vi "Coord list setup-format and values.vi"() -> (13 "Values.Boolean":bool[](array[boolean]), 14 "Keys setup.DBL":T2=[{"key"="Control FPGA.Clock Freq (MHz)", "Save?"=TRUE, "Default"=240.0}, {"key"="DAQ FPGA.Clock Freq (MHz)", "Save?"=TRUE, "Default"=240.0}], 15 "Values.DBL":dbl[](array[numeric]) format="%#_9f", 16 "Keys setup.String":T3=[{"key"="Control FPGA.MAC address", "Save?"=TRUE, "Default"="AABBCCDDEEFF"}, {"key"="DAQ FPGA.Target", "Save?"=TRUE, "Default"="RIO0"}, {"key"="XY Stage.COM port", "Save?"=TRUE, "Default"="COM7"}, {"key"="DAQmx Chan.Pockels Control", "Save?"=TRUE, "Default"=""}, {"key"="DAQmx Chan.Hard Shutter", "Save?"=TRUE, "Default"=""}, {"key"="DAQmx Chan.PMT 1", "Save?"=TRUE, "Default"=""}, {"key"="DAQmx Chan.PMT 2", "Save?"=TRUE, "Default"=""}, {"key"="DAQmx Chan.Encoder Trigger", "Save?"=TRUE, "Default"=""}, {"key"="DAQmx Chan.Optional Trigger 1", "Save?"=TRUE, "Default"=""}, {"key"="DAQmx Chan.Optional Trigger 2", "Save?"=TRUE, "Default"=""}, {"key"="DAQmx Chan.Optional Trigger 3", "Save?"=TRUE, "Default"=""}], 17 "Values.Strings":string[](array[string]), 18 "Keys setup.Boolean":T1, 19 "error out":errorcluster)   [LabVIEW 2017]
uses:
  Typedefs/Ini file interface (String).ctl
  Typedefs/Ini file interface (DBL).ctl
  Typedefs/Ini file interface (Boolean).ctl
  User Interface/Windows/Coordinates list window/Globals/Coord window-Globals.vi
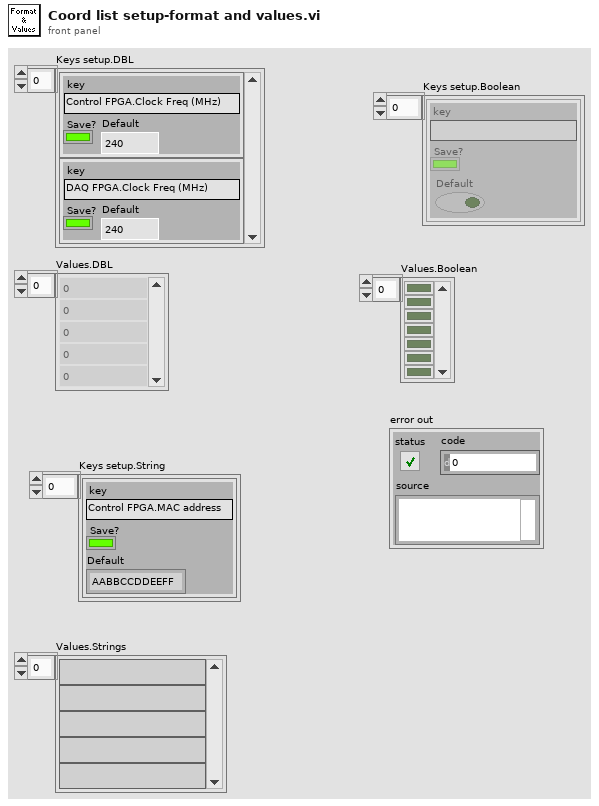
[diagram p1: front panel]
types:
  T1 = typedef "Ini file interface (Boolean).ctl" = cluster{"key":string, "Save?":bool, "Default":bool}[]
  T2 = typedef "Ini file interface (DBL).ctl" = cluster{"key":string, "Save?":bool, "Default":dbl}[]
  T3 = typedef "Ini file interface (String).ctl" = cluster{"key":string, "Save?":bool, "Default":string}[]
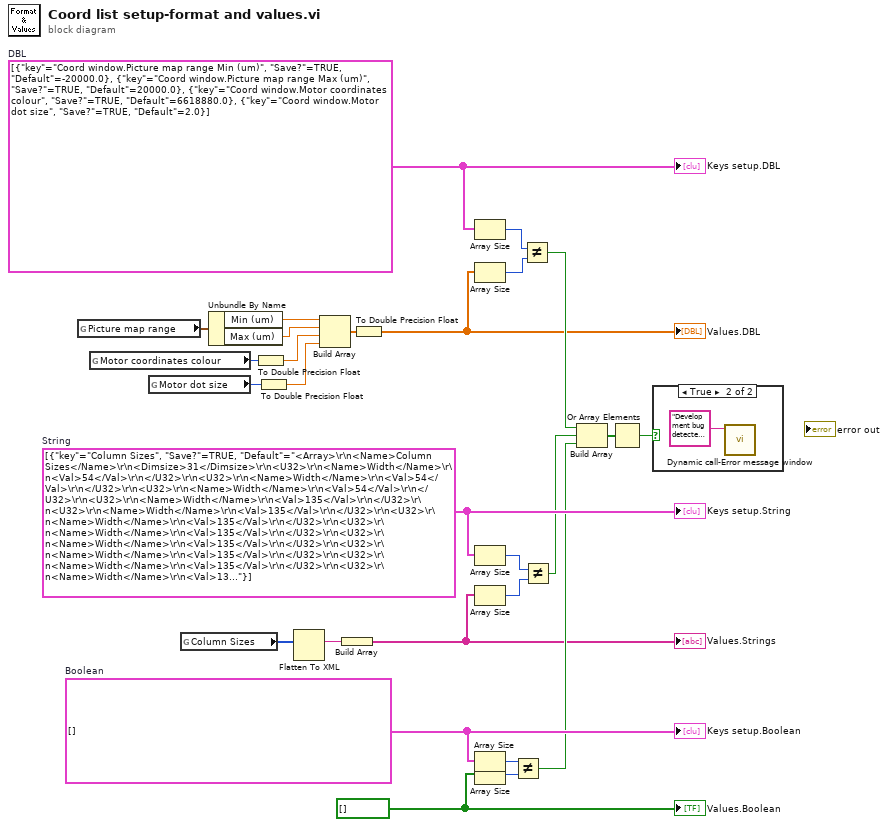
[diagram p0: block diagram]
diagram:
  w13 = bool[] [] ("appended array")
  w25 = T1 []  # Boolean
  w27 = T3 [{"key"="Column Sizes", "Save?"=TRUE, "Default"="<Array>\r\n<Name>Column Sizes</Name>\r\n<Dimsize>31</Dimsize>\r\n<U32>\r\n<Name>Width</Name>\r\n<Val>54</Val>\r\n</U32>\r\n<U32>\r\n<Name>Width</Name>\r\n<Val>54</Val>\r\n</U32>\r\n<U32>\r\n<Name>Width</Name>\r\n<Val>54</Val>\r\n</U32>\r\n<U32>\r\n<Name>Width</Name>\r\n<Val>135</Val>\r\n</U32>\r\n<U32>\r\n<Name>Width</Name>\r\n<Val>135</Val>\r\n</U32>\r\n<U32>\r\n<Name>Width</Name>\r\n<Val>135</Val>\r\n</U32>\r\n<U32>\r\n<Name>Width</Name>\r\n<Val>135</Val>\r\n</U32>\r\n<U32>\r\n<Name>Width</Name>\r\n<Val>135</Val>\r\n</U32>\r\n<U32>\r\n<Name>Width</Name>\r\n<Val>135</Val>\r\n</U32>\r\n<U32>\r\n<Name>Width</Name>\r\n<Val>135</Val>\r\n</U32>\r\n<U32>\r\n<Name>Width</Name>\r\n<Val>135</Val>\r\n</U32>\r\n<U32>\r\n<Name>Width</Name>\r\n<Val>135</Val>\r\n</U32>\r\n<U32>\r\n<Name>Width</Name>\r\n<Val>135</Val>\r\n</U32>\r\n<U32>\r\n<Name>Width</Name>\r\n<Val>135</Val>\r\n</U32>\r\n<U32>\r\n<Name>Width</Name>\r\n<Val>135</Val>\r\n</U32>\r\n<U32>\r\n<Name>Width</Name>\r\n<Val>135</Val>\r\n</U32>\r\n<U32>\r\n<Name>Width</Name>\r\n<Val>135</Val>\r\n</U32>\r\n<U32>\r\n<Name>Width</Name>\r\n<Val>135</Val>\r\n</U32>\r\n<U32>\r\n<Name>Width</Name>\r\n<Val>135</Val>\r\n</U32>\r\n<U32>\r\n<Name>Width</Name>\r\n<Val>135</Val>\r\n</U32>\r\n<U32>\r\n<Name>Width</Name>\r\n<Val>135</Val>\r\n</U32>\r\n<U32>\r\n<Name>Width</Name>\r\n<Val>135</Val>\r\n</U32>\r\n<U32>\r\n<Name>Width</Name>\r\n<Val>135</Val>\r\n</U32>\r\n<U32>\r\n<Name>Width</Name>\r\n<Val>135</Val>\r\n</U32>\r\n<U32>\r\n<Name>Width</Name>\r\n<Val>135</Val>\r\n</U32>\r\n<U32>\r\n<Name>Width</Name>\r\n<Val>135</Val>\r\n</U32>\r\n<U32>\r\n<Name>Width</Name>\r\n<Val>135</Val>\r\n</U32>\r\n<U32>\r\n<Name>Width</Name>\r\n<Val>135</Val>\r\n</U32>\r\n<U32>\r\n<Name>Width</Name>\r\n<Val>135</Val>\r\n</U32>\r\n<U32>\r\n<Name>Width</Name>\r\n<Val>135</Val>\r\n</U32>\r\n<U32>\r\n<Name>Width</Name>\r\n<Val>135</Val>\r\n</U32>\r\n</Array>\r\n"}]  # String
  w26 = T2 [{"key"="Coord window.Picture map range Min (um)", "Save?"=TRUE, "Default"=-20000.0}, {"key"="Coord window.Picture map range Max (um)", "Save?"=TRUE, "Default"=20000.0}, {"key"="Coord window.Motor coordinates colour", "Save?"=TRUE, "Default"=6618880.0}, {"key"="Coord window.Motor dot size", "Save?"=TRUE, "Default"=2.0}]  # DBL
  n1 = global read "Coord window-Globals.vi" "Picture map range"() -> (w11:cluster{"Min (um)":dbl, "Max (um)":dbl})
  n2 = global read "Coord window-Globals.vi" "Motor coordinates colour"() -> (w6:u32)
  n3 = global read "Coord window-Globals.vi" "Motor dot size"() -> (w4:i16)
  n4 = global read "Coord window-Globals.vi" "Column Sizes"() -> (w8:u32[])
  n5 = Unbundle By Name(w11) -> ("Min (um)"=w10:dbl, "Max (um)"=w9:dbl)
  n6 = To Double Precision Float(number=w6) -> (double precision float=w5:dbl)
  n7 = To Double Precision Float(number=w4) -> (double precision float=w3:dbl)
  n8 = Flatten To XML(anything=w8) -> (xml string=w7:string)
  n9 = Build Array(w10, w9, w5, w3) -> (w12:dbl[])
  n10 = Build Array(w7) -> (w1:string[])
  "Values.Strings" <- w1
  n11 = To Double Precision Float(number=w12) -> (double precision float=w2:dbl[])
  "Values.DBL" <- w2
  n12 = Array Size(array=w26) -> (size(s)=w22:i32)
  n13 = Array Size(array=w2) -> (size(s)=w21:i32)
  n14 = Array Size(array=w27) -> (size(s)=w24:i32)
  n15 = Array Size(array=w1) -> (size(s)=w23:i32)
  n16 = Array Size(array=w25) -> (size(s)=w20:i32)
  n17 = Array Size(array=w13) -> (size(s)=w19:i32)
  n18 = Not Equal?(x=w20, y=w19) -> (x != y?=w17:bool)
  n19 = Not Equal?(x=w22, y=w21) -> (x != y?=w15:bool)
  n20 = Not Equal?(x=w24, y=w23) -> (x != y?=w14:bool)
  n21 = Build Array(w15, w14, w17) -> (w18:bool[])
  n22 = Or Array Elements(Boolean array=w18) -> (logical OR=w16:bool)
  n23 = case shown="True" w16 {
    frame False {
    }
    frame True {
      n24 = call "Dynamic call-Error message window.vi"("Error Message"="Development bug detected in the \"Coord list setup-format and values.vi\".\nPlease correct the set up in this VI.") -> ()  [unwired: 10 in, 1 out]
    }
  }
  "Keys setup.String" <- w27
  "Keys setup.DBL" <- w26
  "Keys setup.Boolean" <- w25
  "Values.Boolean" <- w13
